vi "SetActivItemTag.vi"(8 "error in (no error)":errorcluster, 10 "Coords":T1, 11 "ClassDataTree in":refnum<class "ClassDataTree.lvclass">) -> (0 "error out":errorcluster, 3 "ClassDataTree out":refnum<class "ClassDataTree.lvclass">)   [LabVIEW 2010, in "ClassDataTree.lvclass"]
uses:
  ClassDataTree.lvclass
  <vilib>/Utility/miscctls.llb/LVPositionTypeDef.ctl
  <vilib>/Utility/miscctls.llb/LVPoint32TypeDef.ctl
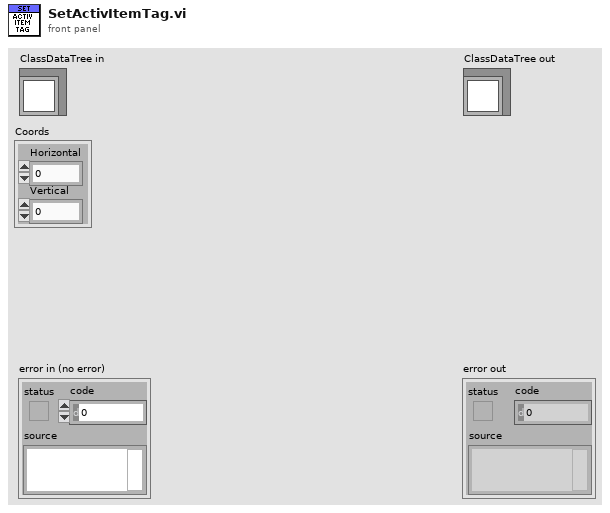
[diagram p1: front panel]
types:
  T1 = typedef "LVPoint32TypeDef.ctl" = cluster{"Horizontal":i32, "Vertical":i32}
  T2 = typedef "LVPositionTypeDef.ctl" = cluster{"Left":i32, "Top":i32}
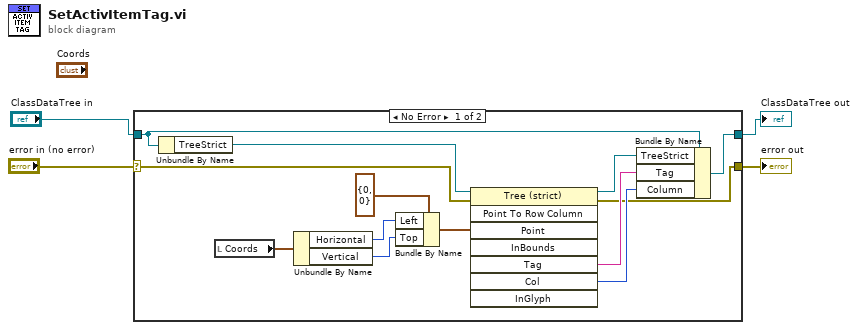
[diagram p0: block diagram]
diagram:
  n1 = case shown="No Error" "error in (no error)" {
    selector: "error in (no error)" -> [w6 w19]
    tunnel: [w5 w19] -> w3
    tunnel: [w12 w18] -> w1
    tunnel: "ClassDataTree in" -> [w16 w18]
    frame No Error {
      n2 = Unbundle By Name(w16) -> ("TreeStrict"=w17:refnum<vi>)
      n3 = local read "Coords"() -> (w10:T1)
      n4 = Unbundle By Name(w10) -> ("Horizontal"=w9:i32, "Vertical"=w8:i32)
      n5 = Bundle By Name(cluster=T2 {"Left"=0, "Top"=0} ("Point"), "Left"=w9, "Top"=w8) -> (w7:T2)
      n6 = invoke class="Tree (strict)" method="Point To Row Column"(reference=w17, error in=w6, "Point"=w7) -> (reference out=w15:refnum<vi>, error out=w5:errorcluster, "Tag"=w14:string, "Col"=w13:i32)  [unwired: 5 in, 4 out]
      n7 = Bundle By Name(cluster=w16, "TreeStrict"=w15, "Tag"=w14, "Column"=w13) -> (w12:refnum<class "ClassDataTree.lvclass">)
    }
    frame Error {
    }
  }
  "error out" <- w3
  "ClassDataTree out" <- w1
